vi "custom commands.vi"(8 "error in (no error)":errorcluster {"code" format="%.0x"}, 9 "format string":string="INITORG", 10 "Device Number (1)":i32=1, 11 "VISA Resource Name":refnum<visa-resource-name>) -> (0 "error out":errorcluster {"code" format="%.0x"}, 2 "Result":string, 3 "VISA Resource Name Out":refnum<visa-resource-name>)   [LabVIEW 2020]
uses:
  Drivers/Olympus IX BX Series/Olympus IX BX Series.lvlib
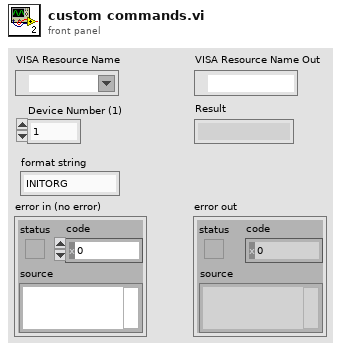
[diagram p1: front panel]
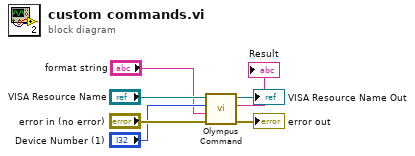
[diagram p0: block diagram]
diagram:
  n1 = call "Olympus Command.vi"("error in (no error)"="error in (no error)", "Command string"="format string", "Device Number (1)"="Device Number (1)", "VISA Resource Name"="VISA Resource Name") -> ("error out"=→"error out":errorcluster, "Result"=→"Result":string, "VISA Resource Name Out"=→"VISA Resource Name Out":refnum<visa-resource-name>)  [unwired: 5 in]
